vi "Toolbar Set Button Image (Vi).vi"(0 "Display State In":T2={"Buttons Displayed"=0, "Button States"=[], "Button Size"=0, "Button Style"=enum."Classic", "Active Button"=0, "Force Regen?"=FALSE, "Tip String Ref"=refnum}, 1 "State":T1, 5 "Button Index":i32, 7 "VI Refnum":refnum<vi>, 9 "Container State":T4, 11 "error in (no error)":errorcluster) -> (4 "Display State Out":T2={"Buttons Displayed"=0, "Button States"=[], "Button Size"=0, "Button Style"=enum."Classic", "Active Button"=0, "Force Regen?"=FALSE, "Tip String Ref"=refnum}, 15 "error out":errorcluster)   [LabVIEW 2012, in "Toolbar.xctl"]
doc: "Sets the toolbar button image for a specific state using the icon of a VI"
uses:
  Toolbar.xctl
  <vilib>/_xctls/Container State.ctl
  Toolbar State.ctl
  Button_Class/Button.lvclass
  Button_Class/Type Defs/Button Style.ctl
  Button_Class/Type Defs/Button Status.ctl
  <vilib>/_xctls/XControlSupport.lvlib
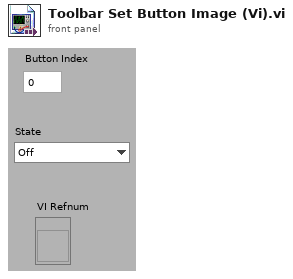
[diagram p1: front panel]
types:
  T1 = typedef "Button.lvclass/Button Status.ctl" = enum16{"Off", "Hover", "On", "Disabled"}
  T2 = typedef "Toolbar.xctl/Toolbar State.ctl" = cluster{"Buttons Displayed":i32, "Button States":refnum<class "Button.lvclass">[], "Button Size":i32, "Button Style":T3, "Active Button":i32, "Force Regen?":bool, "Tip String Ref":refnum<vi>}
  T3 = typedef "Button.lvclass/Button Style.ctl" = enum16{"System", "Modern", "Classic", "Rounded", "Silver", "Ni Theme", "Metallic"}
  T4 = typedef "XControlSupport.lvlib/Container State.ctl" = cluster{"Indicator?":bool, "Run Mode?":bool, " Refnum":refnum<vi>}
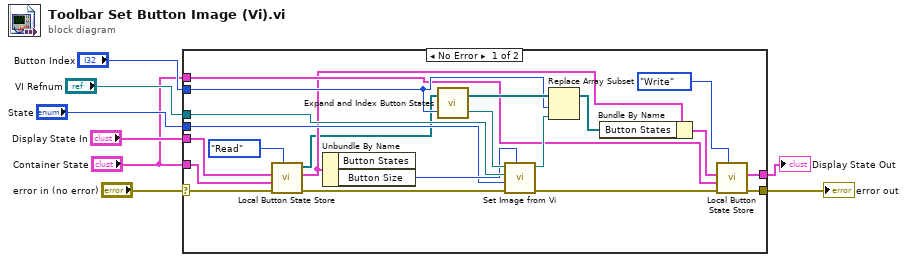
[diagram p0: block diagram]
diagram:
  n1 = case shown="No Error" "error in (no error)" {
    selector: "error in (no error)" -> [w22 w30]
    tunnel: "Display State In" -> [w11 w31]
    tunnel: [w14 w31] -> w3
    tunnel: [w16 w30] -> w2
    tunnel: "Button Index" -> [w28 _]
    tunnel: "State" -> [w23 _]
    tunnel: "VI Refnum" -> [w25 _]
    tunnel: "Container State" -> [w13 _]
    tunnel: "Container State" -> [w12 _]
    frame No Error {
      n2 = call "Local Button State Store.vi"("Operation"=enum16{"Read", "Write"}."Read", "error in (no error)"=w22, "Container State"=w12, "Display State In"=w11) -> ("error out"=w21:errorcluster, "Display State Out"=w10:T2, "Button States"=w9:refnum<class "Button.lvclass">[])  [unwired: 5 out]
      n3 = Unbundle By Name(w10) -> ("Button Size"=w24:i32)  [unwired: 1 out]
      n4 = call "Expand and Index Button States.vi"("Button Index"=w28, "Button States"=w9) -> ("Button.lvclass"=w27:refnum<class "Button.lvclass">, "Button States Out"=w29:refnum<class "Button.lvclass">[])
      n5 = call-dynamic "Set Image from Vi.vi"("Button Size"=w24, "error in (no error)"=w21, "State"=w23, "VI Refnum"=w25, "Button in"=w27) -> ("error out"=w17:errorcluster, "Button out"=w26:refnum<class "Button.lvclass">)  [unwired: 1 in, 4 out]
      n6 = Replace Array Subset(array=w29, new element=w26, index=w28) -> (w19:refnum<class "Button.lvclass">[])
      n7 = Bundle By Name(cluster=w10, "Button States"=w19) -> (w15:T2)
      n8 = call "Local Button State Store.vi"("Operation"=enum16{"Read", "Write"}."Write", "error in (no error)"=w17, "Container State"=w13, "Display State In"=w15) -> ("error out"=w16:errorcluster, "Display State Out"=w14:T2)  [unwired: 1 in, 5 out]
    }
    frame Error {
    }
  }
  "Display State Out" <- w3
  "error out" <- w2
